vi "parseQuickKey.vi"(0 "VISA resource name":refnum<visa-resource-name>, 1 "write buffer":string="®\b", 3 "y":i32=2, 4 "x":i32, 5 "error in (no error)":errorcluster) -> (14 "lengthString":i32, 15 "KeyCodeName":string[](array[string]), 16 "BinaryString":string, 18 "No Keys":bool, 19 "error out":errorcluster)   [LabVIEW 2018]
uses:
  Global_usbComm.vi
panel:
  out "lo":string
  out "hi":string
  out "True Array":string[](array[string])
  out "False Array":string[](array[string])
  out "byte integer string":string[](array[string])
  out "String to Array":string[](array[string])
  # "y-selector Key Table\nMPH-0\nKPH-1\nINC-2\nRES-3\nGEA-4"
  # "Array, y, x - console - function\ntrue,2,16 - 28717 - incline\ntrue,1,0 - speed\ntrue, 2, 16 - 50915 - incline\ntrue, 0, 0 - speed\ntrue, 3, 0 - 05918 - resistance\ntrue, 2, 16 -78717 - incline\ntrue, 1, 0 - speed\ntrue, 3, 0 - 55918 - resitance\ntrue, 2, 0 - 19119 - incline\ntrue, 0, 0 -speed"
  # "x-selector Bit Offset\nspeed-0\nincline-0\nresistance-0\ngear-0"
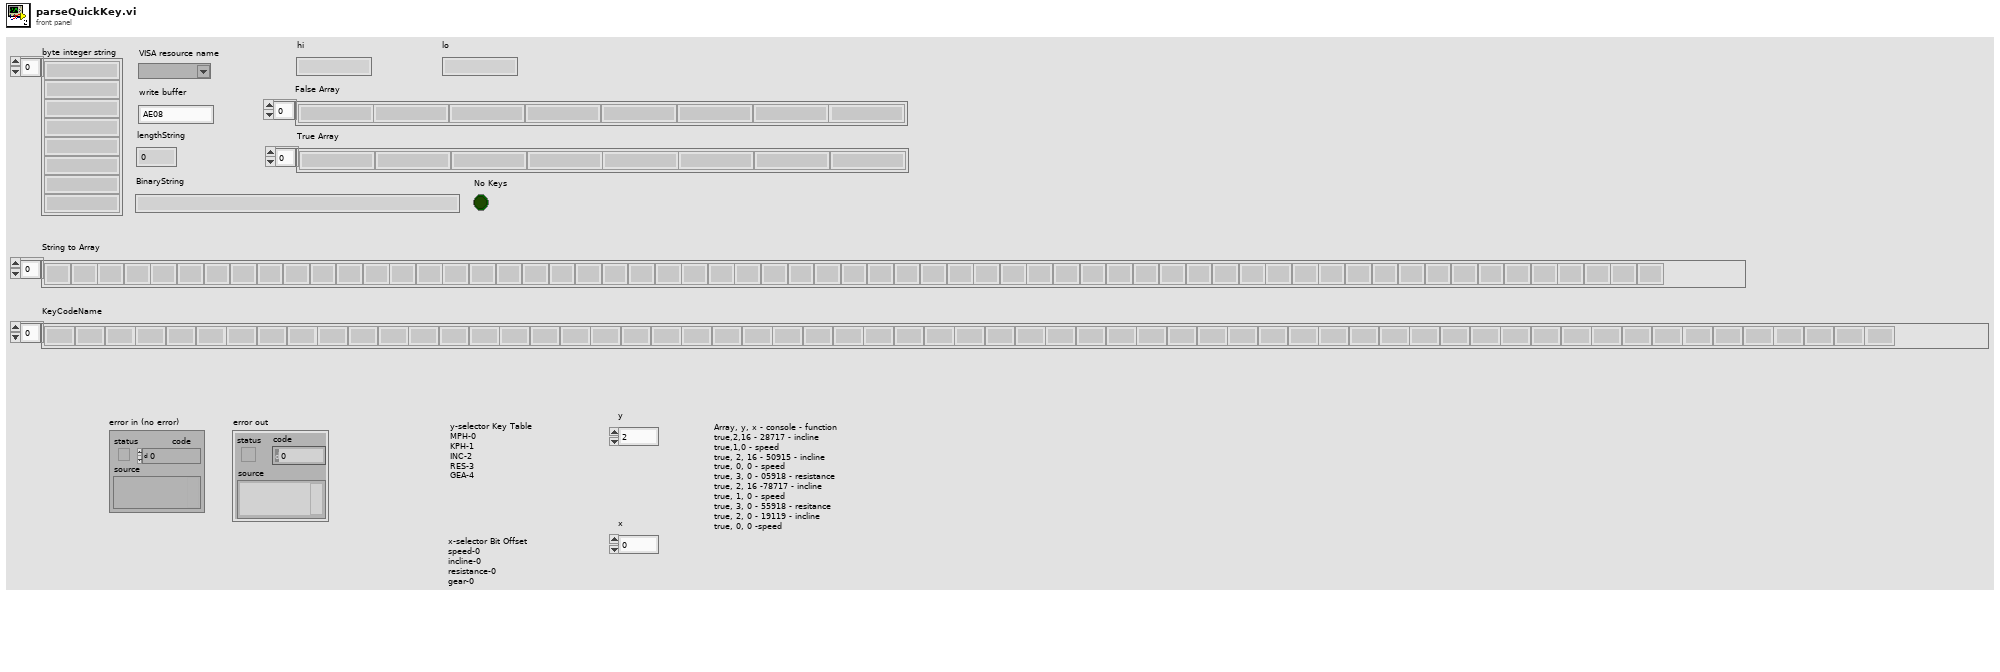
[diagram p1: front panel]
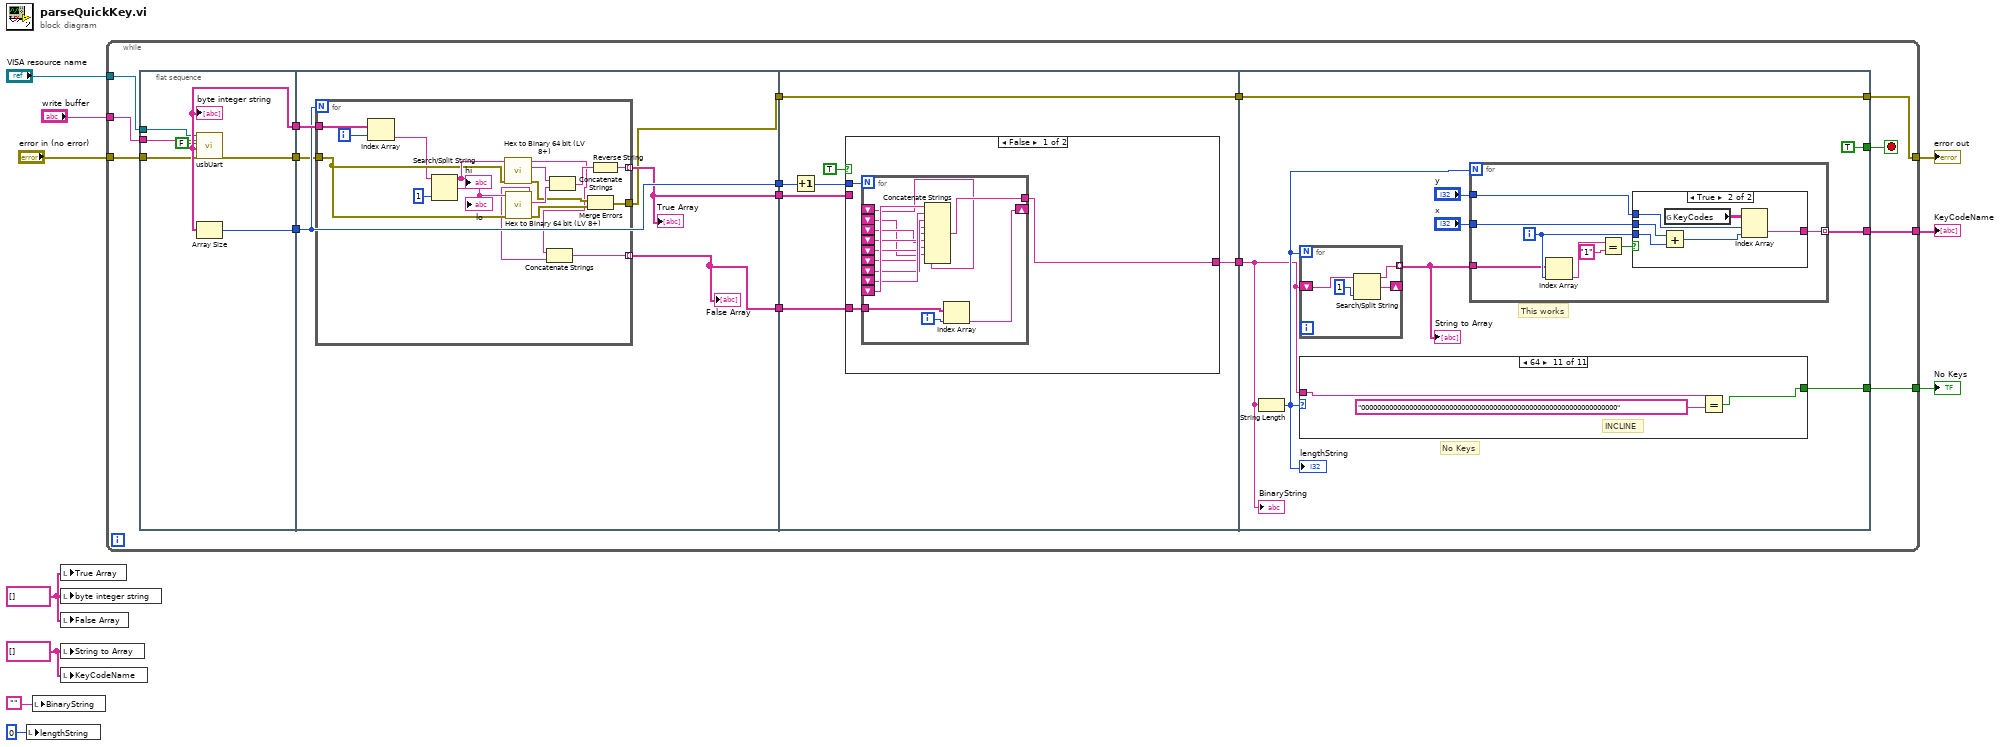
[diagram p0: block diagram]
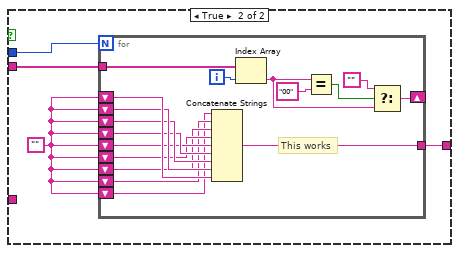
[diagram p2: hidden frame]
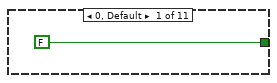
[diagram p3: hidden frame]
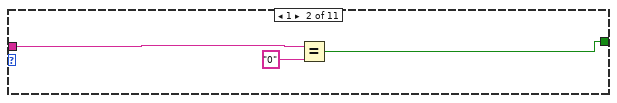
[diagram p4: hidden frame]
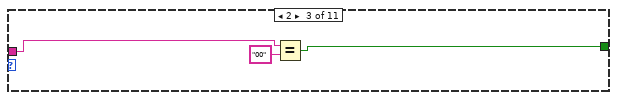
[diagram p5: hidden frame]
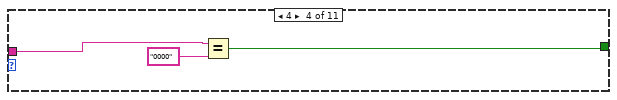
[diagram p6: hidden frame]
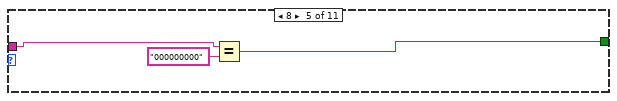
[diagram p7: hidden frame]
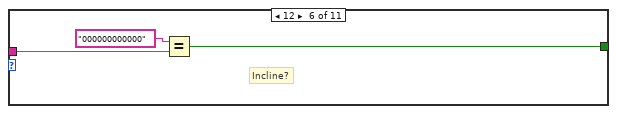
[diagram p8: hidden frame]
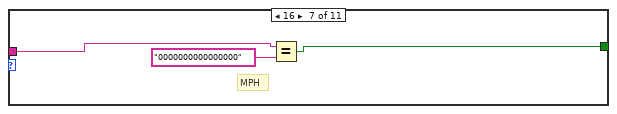
[diagram p9: hidden frame]
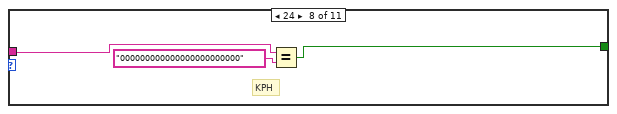
[diagram p10: hidden frame]
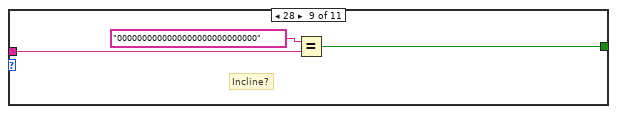
[diagram p11: hidden frame]
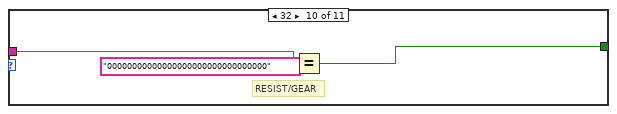
[diagram p12: hidden frame]
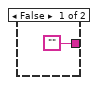
[diagram p13: hidden frame]
diagram:
  w4 = string[] [] ("String to Array")
  w6 = string[] []
  n1 = local write "lengthString"(0 ("lengthString")) -> ()
  n2 = local write "BinaryString"("") -> ()
  n3 = local write "True Array"(w6) -> ()
  n4 = local write "byte integer string"(w6) -> ()
  n5 = local write "False Array"(w6) -> ()
  n6 = local write "String to Array"(w4) -> ()
  n7 = local write "KeyCodeName"(w4) -> ()
  n8 = while {
    tunnel: "VISA resource name" -> [w20]
    tunnel: [w18] -> w7
    tunnel: "write buffer" -> [w16]
    tunnel: [w15] -> w1
    tunnel: "error in (no error)" -> [w19]
    tunnel: [w12] -> w10
    stop <- w17 stop-if-true
    n9 = flat-sequence {
      tunnel: [w33] -> w26
      tunnel: [w31] -> w25
      tunnel: [w32] -> w24
      tunnel: w20 -> [w30]
      tunnel: w19 -> [w29]
      tunnel: w16 -> [w28]
      tunnel: [w38] -> w23
      tunnel: [w36] -> w22
      tunnel: w26 -> [w39]
      tunnel: w25 -> [w38]
      tunnel: w24 -> [w37]
      tunnel: [w34] -> w14
      tunnel: [w35] -> w13
      tunnel: w23 -> [w63]
      tunnel: w22 -> [w61]
      tunnel: [w60] -> w21
      tunnel: w14 -> [w58]
      tunnel: w13 -> [w57]
      tunnel: [w57] -> w11
      tunnel: w21 -> [w103]
      tunnel: [w106] -> w18
      tunnel: [TRUE] -> w17
      tunnel: [w102] -> w15
      tunnel: [w101] -> w12
      tunnel: w11 -> [w101]
      frame #0 {
        n10 = call "usbUart.vi"("VISA resource name"=w30, "write buffer"=w28, "sdFeature"=FALSE, "error in (no error)"=w29) -> ("byte integer string"=w33:string[], "error out"=w32:errorcluster)  [unwired: 14 out]
        "byte integer string" <- w33
        n11 = Array Size(array=w33) -> (size(s)=w31:i32)
      }
      frame #1 {
        n12 = for {
          N: w38 -> [_]
          tunnel: w39 -> [w56]
          tunnel: [w54] -> w36 mode=indexing
          tunnel: w37 -> [w46]
          tunnel: [w45] -> w35
          tunnel: [w40] -> w34 mode=indexing
          i -> [w55]
          n13 = Index Array(array=w56, index=w55) -> (element=w43:string)
          n14 = Search/Split String(string=w43, offset (0)=1) -> (substring before match=w53:string, match + rest of string=w52:string)  [unwired: 1 in, 1 out]
          "hi" <- w53
          "lo" <- w52
          n15 = call "Hex to Binary 64 bit (LV 8+).vi"("error in (no error)"=w46, "Hexadecimal String"=w53) -> ("error out"=w48:errorcluster, "add 0's' String"=w50:string, "Binary String"=w42:string)  [unwired: 5 in]
          n16 = call "Hex to Binary 64 bit (LV 8+).vi"("error in (no error)"=w46, "Hexadecimal String"=w52) -> ("error out"=w47:errorcluster, "add 0's' String"=w49:string, "Binary String"=w41:string)  [unwired: 5 in]
          n17 = Concatenate Strings(w42, w41) -> (w40:string)
          n18 = Concatenate Strings(w50, w49) -> (w51:string)
          n19 = Merge Errors(w48, w47) -> (w45:errorcluster)
          n20 = Reverse String(1:w51) -> (0:w54:string)
        }
        "False Array" <- w34
        "True Array" <- w36
      }
      frame #2 {
        n21 = Increment(x=w63) -> (x+1=w62:i32)
        n22 = case shown="False" TRUE ("Array") {
          tunnel: [w66 w83] -> w60
          tunnel: w62 -> [w65 w82]
          tunnel: w61 -> [_ w81]
          tunnel: w58 -> [w64 _]
          frame False {
            n23 = for {
              N: w65 -> [_]
              shift-right: [w77] -> _
              shift-left: _ -> [w67]
              shift-left: _ -> [w68]
              shift-left: _ -> [w69]
              shift-left: _ -> [w70]
              shift-left: _ -> [w71]
              shift-left: _ -> [w72]
              shift-left: _ -> [w73]
              shift-left: _ -> [w74]
              shift-left: _ -> [w75]
              tunnel: [w78] -> w66
              tunnel: w64 -> [w76]
              i -> [w79]
              n24 = Concatenate Strings(w75, w74, w73, w72, w71, w70, w69, w68, w67) -> (w78:string)
              n25 = Index Array(array=w76, index=w79) -> (element=w77:string)
            }
          }
          frame True {
            w80 = ""
            n26 = for {
              N: w82 -> [_]
              shift-right: [w96] -> _
              shift-left: w80 -> [w95]
              shift-left: w80 -> [w94]
              shift-left: w80 -> [w93]
              shift-left: w80 -> [w92]
              shift-left: w80 -> [w91]
              shift-left: w80 -> [w90]
              shift-left: w80 -> [w89]
              shift-left: w80 -> [w88]
              shift-left: w80 -> [w87]
              tunnel: [w86] -> w83
              tunnel: w81 -> [w85]
              i -> [w100]
              # "This works"
              n27 = Concatenate Strings(w87, w88, w89, w90, w91, w92, w93, w94, w95) -> (w86:string)
              n28 = Index Array(array=w85, index=w100) -> (element=w84:string)
              n29 = Equal?(x=w84, y="00") -> (x = y?=w98:bool)
              n30 = Select(t="", s=w98, f=w84) -> (s? t:f=w96:string)
            }
          }
        }
      }
      frame #3 {
        # "No Keys"
        # "This works"
        n31 = String Length(string=w103) -> (length=w104:i32)
        "lengthString" <- w104
        n32 = for {
          N: w104 -> [_]
          shift-right: [w159] -> _
          shift-left: w103 -> [w158]
          tunnel: [w157] -> w107 mode=indexing
          n33 = Search/Split String(string=w158, offset (0)=1) -> (substring before match=w157:string, match + rest of string=w159:string)  [unwired: 1 in, 1 out]
        }
        "String to Array" <- w107
        n34 = case shown="64" w104 {
          tunnel: w103 -> [_ w112 w115 w118 w121 w125 w127 w130 w133 w135 w139]
          tunnel: [FALSE w111 w114 w117 w120 w123 w126 w129 w134 w136 w138] -> w102
          frame 0, Default {
          }
          frame 1 {
            n35 = Equal?(x=w112, y="0") -> (x = y?=w111:bool)
          }
          frame 2 {
            n36 = Equal?(x=w115, y="00") -> (x = y?=w114:bool)
          }
          frame 4 {
            n37 = Equal?(x=w118, y="0000") -> (x = y?=w117:bool)
          }
          frame 8 {
            n38 = Equal?(x=w121, y="000000000") -> (x = y?=w120:bool)
          }
          frame 12 {
            # "Incline?"
            n39 = Equal?(x="000000000000", y=w125) -> (x = y?=w123:bool)
          }
          frame 16 {
            # "MPH"
            n40 = Equal?(x=w127, y="0000000000000000") -> (x = y?=w126:bool)
          }
          frame 24 {
            # "KPH"
            n41 = Equal?(x=w130, y="000000000000000000000000") -> (x = y?=w129:bool)
          }
          frame 28 {
            # "Incline?"
            n42 = Equal?(x="0000000000000000000000000000", y=w133) -> (x = y?=w134:bool)
          }
          frame 32 {
            # "RESIST/GEAR"
            n43 = Equal?(x=w135, y="00000000000000000000000000000000") -> (x = y?=w136:bool)
          }
          frame 64 {
            # "INCLINE"
            n44 = Equal?(x=w139, y="0000000000000000000000000000000000000000000000000000000000000000") -> (x = y?=w138:bool)
          }
        }
        n45 = for {
          N: w104 -> [_]
          tunnel: [w145] -> w106 mode=indexing
          tunnel: w107 -> [w144]
          tunnel: "x" -> [w142]
          tunnel: "y" -> [w141]
          i -> [w146]
          n46 = Index Array(array=w144, index=w146) -> (element=w143:string)
          n47 = Equal?(x=w143, y="1") -> (x = y?=w147:bool)
          n48 = case shown="True" w147 {
            tunnel: w146 -> [_ w153]
            tunnel: ["" w154] -> w145
            tunnel: w142 -> [_ w151]
            tunnel: w141 -> [_ w150]
            frame False {
            }
            frame True {
              n49 = Add(x=w151, y=w153) -> (x+y=w152:i32)
              n50 = global read "Global_usbComm.vi" "KeyCodes"() -> (w155:string[][])
              n51 = Index Array(array=w155, index (row)=w150, index (col)=w152) -> (element=w154:string)
            }
          }
        }
        "BinaryString" <- w103
      }
    }
  }
  "error out" <- w10
  "KeyCodeName" <- w7
  "No Keys" <- w1
